vi "Get Ingredients.vi"(8 "error in (no error)":errorcluster, 11 "Simple Circuit in":refnum<class "Simple Circuit.lvclass">) -> (0 "error out":errorcluster, 2 "Ingredients":T1[](array[typedef]), 3 "Simple Circuit out":refnum<class "Simple Circuit.lvclass">)   [LabVIEW 2020, in "Simple Circuit.lvclass"]
uses:
  Simple Circuit.lvclass
  Item/Ingredient.ctl
  Item/Item.lvclass
  Electronic Parts/Electronic Parts.lvclass
  C:/dev/LabVIEW/Good Company Calc/Item/Item.lvclass
  Circuit Board/Circuit Board.lvclass
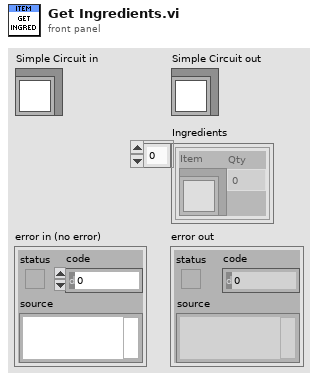
[diagram p1: front panel]
types:
  T1 = typedef "Item.lvclass/Ingredient.ctl" = cluster{"Item":refnum<class "Item.lvclass">, "Qty":dbl}
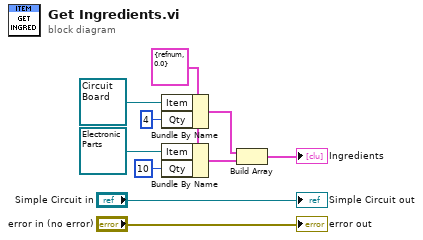
[diagram p0: block diagram]
diagram:
  w6 = T1 {"Item"=refnum, "Qty"=0.0} ("Ingredient")
  n1 = Bundle By Name(cluster=w6, "Item"=refnum<class "Circuit Board.lvclass"> refnum ("Circuit Board.lvclass"), "Qty"=4) -> (w4:T1)
  n2 = Bundle By Name(cluster=w6, "Item"=refnum<class "Electronic Parts.lvclass"> refnum ("Electronic Parts.lvclass"), "Qty"=10) -> (w5:T1)
  n3 = Build Array(w4, w5) -> (→"Ingredients":T1[])
  "error out" <- "error in (no error)"
  "Simple Circuit out" <- "Simple Circuit in"
